vi "RelayPosition to RelayAction.vi"(10 "position":T1=11 items=["Open"=10, "Closed"=11]) -> (2 "action":T2=21 caption="relay action" items=["CloseRelay"=21, "OpenRelay"=20])   [LabVIEW 2016, in "SLSC Switch.lvlib" / "slscsl.lvclass"]
uses:
  slscsl.lvclass
  RelayAction.ctl
  RelayPosition.ctl
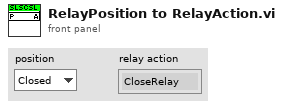
[diagram p1: front panel]
types:
  T1 = typedef "SLSC Switch.lvlib/slscsl.lvclass/RelayPosition.ctl" = i32
  T2 = typedef "SLSC Switch.lvlib/slscsl.lvclass/RelayAction.ctl" = u32
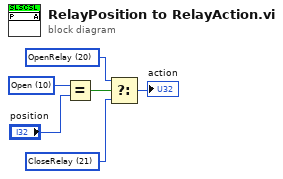
[diagram p0: block diagram]
diagram:
  w1 = T2 21 items=["CloseRelay"=21, "OpenRelay"=20] ("RelayAction")
  w2 = T2 20 items=["CloseRelay"=21, "OpenRelay"=20] ("RelayAction")
  w4 = T1 10 items=["Open"=10, "Closed"=11] ("x")
  n1 = Equal?(x=w4, y="position") -> (x = y?=w5:bool)
  n2 = Select(t=w2, s=w5, f=w1) -> (s? t:f=→"action":T2)
